vi "INI_driver.vi"(5 "create file if necessary (T)":bool=TRUE, 6 "Enum":T1(ring), 7 "instrument file path":path, 8 "error in (no error)":errorcluster, 9 "Value_in":string[](array[string]), 10 "Section":string, 11 "Key_name":string[](array[string])) -> (0 "error out":errorcluster, 1 "section names":string[](array[string]), 2 "Values out":string[](array[string]), 3 "key names":string[](array[string]))   [LabVIEW 2024, in "Launcher_DTU.lvlib"]
uses:
  Launcher_DTU.lvlib
  <vilib>/Utility/config.llb/Read Key (String).vi
  <vilib>/Utility/config.llb/Write Key (String).vi
  <vilib>/Utility/config.llb/NI_LVConfig.lvlib
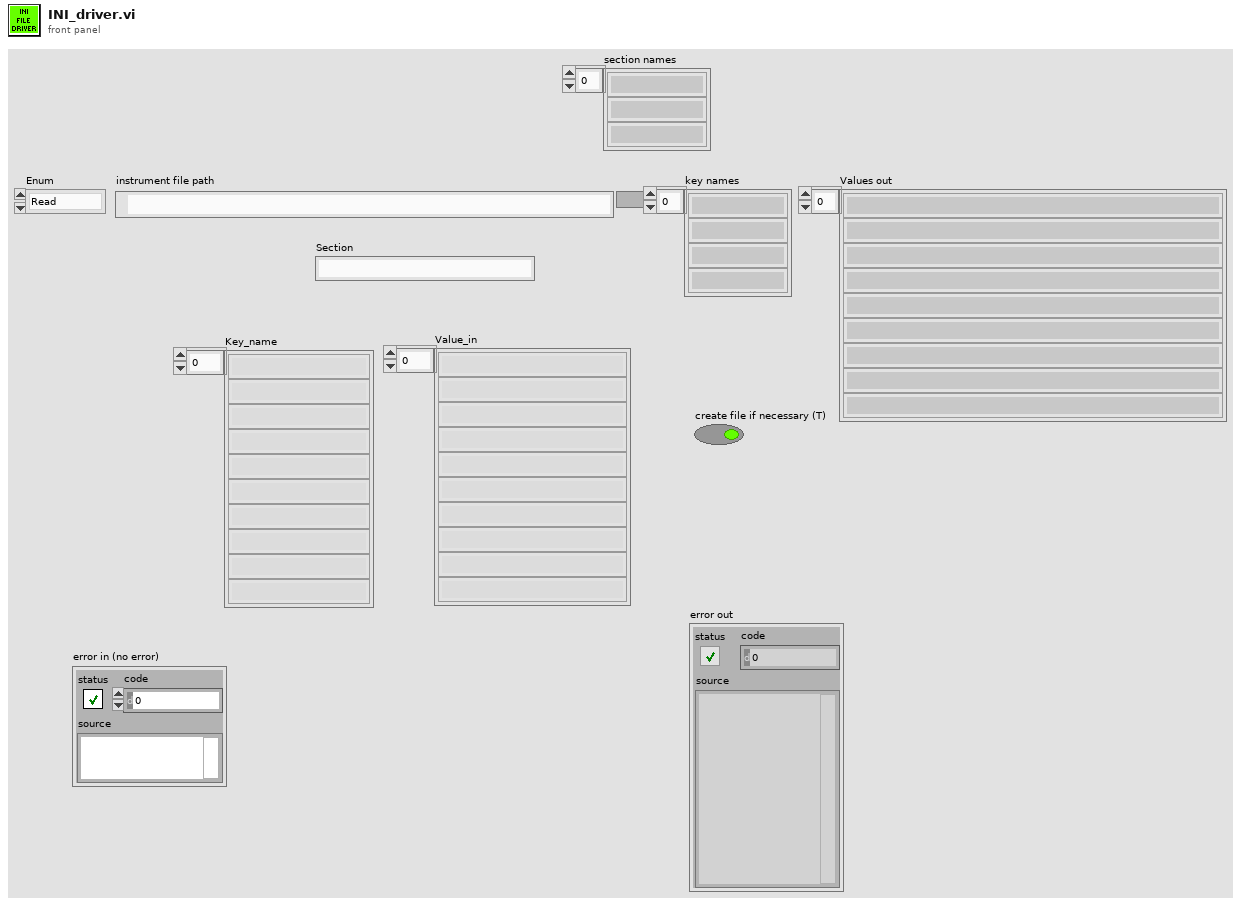
[diagram p1: front panel]
types:
  T1 = enum16{"Read", "Write", "All_sections", "All_values", "Remove key&section"}
  T2 = typedef "NI_LVConfig.lvlib/Config Data RefNum.ctl" = refnum<k1>
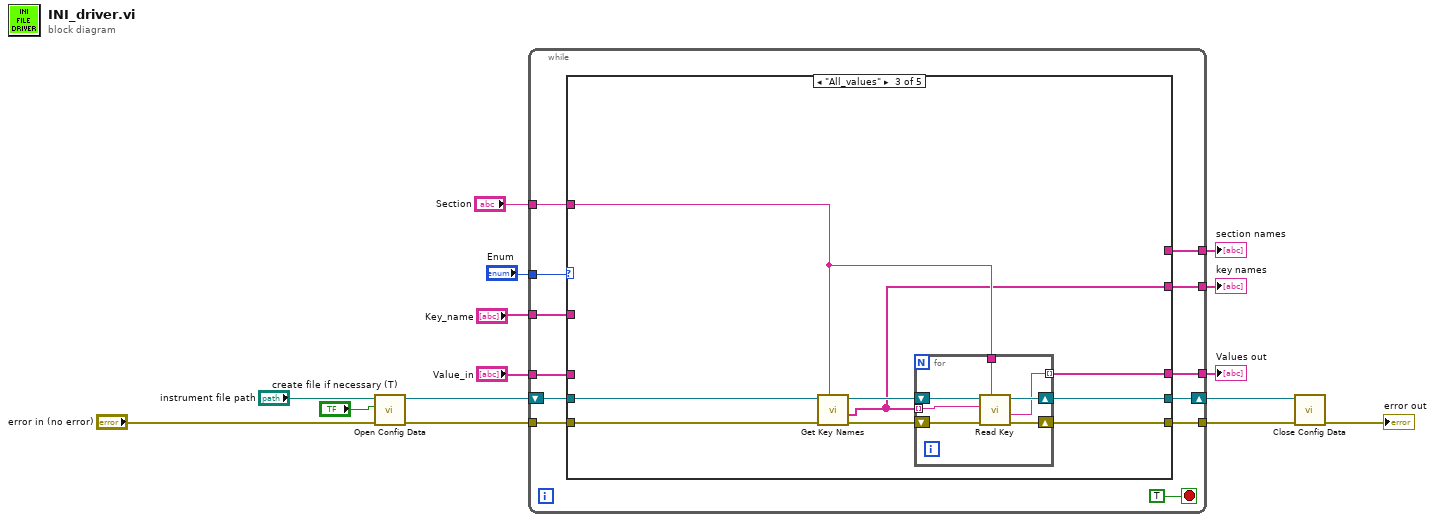
[diagram p0: block diagram]
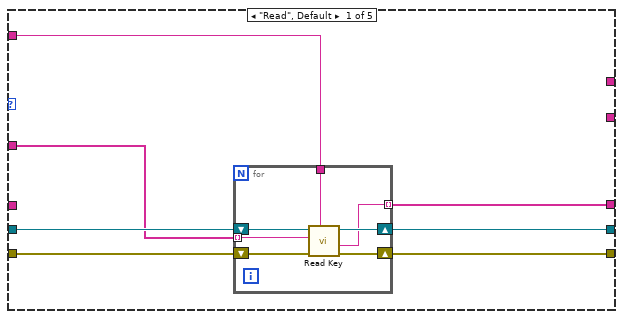
[diagram p2: hidden frame]
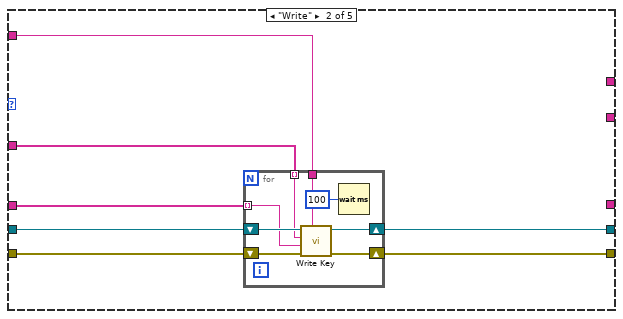
[diagram p3: hidden frame]
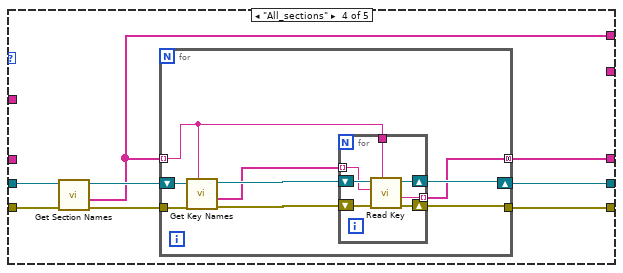
[diagram p4: hidden frame]
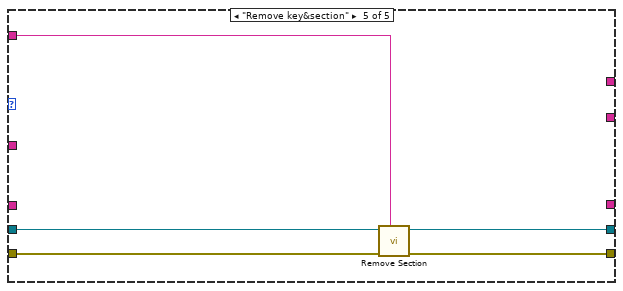
[diagram p5: hidden frame]
diagram:
  n1 = call <vilib>:"Open Config Data.vi"("error in (no error)"="error in (no error)", "create file if necessary (T)"="create file if necessary (T)", "configuration file path"="instrument file path") -> ("error out"=w13:errorcluster, "refnum"=w12:T2)  [unwired: 6 in, 1 out]
  n2 = while {
    tunnel: w13 -> [w27]
    tunnel: [w26] -> w11
    tunnel: "Section" -> [w22]
    tunnel: "Key_name" -> [w21]
    tunnel: "Value_in" -> [w20]
    tunnel: [w19] -> w1
    tunnel: "Enum" -> [w18]
    tunnel: [w17] -> w3
    tunnel: [w16] -> w2
    shift-right: [w23] -> w9
    shift-left: w12 -> [w25]
    stop <- TRUE stop-if-true
    n3 = case shown="\"All_values\"" w18 {
      tunnel: w27 -> [w34 w48 w65 w80 w100]
      tunnel: [w33 w47 w62 w77 w101] -> w26
      tunnel: w25 -> [w32 w46 w63 w79 w98]
      tunnel: [w31 w45 w60 w74 w97] -> w23
      tunnel: w22 -> [w30 w44 w59 _ w99]
      tunnel: w21 -> [w29 w43 _ _ _]
      tunnel: w20 -> [_ w42 _ _ _]
      tunnel: [w28 _ w58 w75 _] -> w19
      tunnel: [_ _ w57 _ _] -> w17
      tunnel: [_ _ _ w73 _] -> w16
      frame "Read", Default {
        n4 = for {
          tunnel: w30 -> [w37]
          tunnel: w29 -> [w36] mode=indexing
          shift-right: [w40] -> w33
          shift-left: w34 -> [w41]
          shift-right: [w38] -> w31
          shift-left: w32 -> [w39]
          tunnel: [w35] -> w28 mode=indexing
          n5 = call-poly <vilib>:"Read Key.vi"("section"=w37, "error in (no error)"=w41, "key"=w36, "refnum"=w39) -> ("error out"=w40:errorcluster, "value"=w35:string, "refnum out"=w38:T2)  [unwired: 4 in, 1 out]
        }
      }
      frame "Write" {
        n6 = for {
          tunnel: w44 -> [w52]
          shift-right: [w55] -> w47
          shift-left: w48 -> [w56]
          shift-right: [w53] -> w45
          shift-left: w46 -> [w54]
          tunnel: w43 -> [w51] mode=indexing
          tunnel: w42 -> [w50] mode=indexing
          n7 = call-poly <vilib>:"Write Key.vi"("section"=w52, "error in (no error)"=w56, "value"=w50, "key"=w51, "refnum"=w54) -> ("error out"=w55:errorcluster, "refnum out"=w53:T2)  [unwired: 4 in, 1 out]
          n8 = Wait (ms)(milliseconds to wait=u32 100) -> ()  [unwired: 1 out]
        }
      }
      frame "All_values" {
        n9 = call <vilib>:"Get Key Names.vi"("section"=w59, "error in (no error)"=w65, "refnum"=w63) -> ("error out"=w64:errorcluster, "key names"=w57:string[], "refnum out"=w61:T2)  [unwired: 5 in, 1 out]
        n10 = for {
          shift-right: [w71] -> w62
          shift-left: w64 -> [w72]
          shift-right: [w69] -> w60
          shift-left: w61 -> [w70]
          tunnel: w57 -> [w68] mode=indexing
          tunnel: w59 -> [w67]
          tunnel: [w66] -> w58 mode=indexing
          n11 = call-poly <vilib>:"Read Key.vi"("section"=w67, "error in (no error)"=w72, "key"=w68, "refnum"=w70) -> ("error out"=w71:errorcluster, "value"=w66:string, "refnum out"=w69:T2)  [unwired: 4 in, 1 out]
        }
      }
      frame "All_sections" {
        n12 = call <vilib>:"Get Section Names.vi"("error in (no error)"=w80, "refnum"=w79) -> ("error out"=w78:errorcluster, "section names"=w73:string[], "refnum out"=w76:T2)  [unwired: 7 in]
        n13 = for {
          tunnel: w78 -> [w89]
          tunnel: [w84] -> w77
          tunnel: w73 -> [w82] mode=indexing
          shift-right: [w85] -> w74
          shift-left: w76 -> [w88]
          tunnel: [w81] -> w75 mode=concatenating
          n14 = call <vilib>:"Get Key Names.vi"("section"=w82, "error in (no error)"=w89, "refnum"=w88) -> ("error out"=w87:errorcluster, "key names"=w83:string[], "refnum out"=w86:T2)  [unwired: 5 in, 1 out]
          n15 = for {
            tunnel: w83 -> [w92] mode=indexing
            shift-right: [w93] -> w84
            shift-left: w87 -> [w96]
            shift-right: [w94] -> w85
            shift-left: w86 -> [w95]
            tunnel: [w91] -> w81 mode=indexing
            tunnel: w82 -> [w90]
            n16 = call-poly <vilib>:"Read Key.vi"("section"=w90, "error in (no error)"=w96, "key"=w92, "refnum"=w95) -> ("error out"=w93:errorcluster, "value"=w91:string, "refnum out"=w94:T2)  [unwired: 4 in, 1 out]
          }
        }
      }
      frame "Remove key&section" {
        n17 = call <vilib>:"Remove Section.vi"("section"=w99, "error in (no error)"=w100, "refnum"=w98) -> ("error out"=w101:errorcluster, "refnum out"=w97:T2)  [unwired: 6 in, 1 out]
      }
    }
  }
  "Values out" <- w1
  "key names" <- w3
  "section names" <- w2
  n18 = call <vilib>:"Close Config Data.vi"("error in (no error)"=w11, "refnum"=w9) -> ("error out"=→"error out":errorcluster)  [unwired: 8 in, 1 out]
